vi "StageControl.vi"() -> ()   [LabVIEW 2013]
panel:
  in  "ESP Port":refnum<visa-resource-name>="COM4"
  out "Location Matrix":string[][](array[string])=[["N.D.\r\n", "N.D.\r\n", "N.D.\r\n"], ["N.D.\r\n", "N.D.\r\n", "N.D.\r\n"], ["N.D.\r\n", "N.D.\r\n", "N.D.\r\n"], ["N.D.\r\n", "N.D.\r\n", "N.D.\r\n"]]
  in  "Capture Locations":i32(listbox)=2
  in  "?":cluster{"x":string, "y":string, "z":string}={"x"="N.D.\r\n", "y"="N.D.\r\n", "z"="N.D.\r\n"}
  out "Location path":path=path "C:/Users/Fleezers/Desktop/UHR-Fleezers Instrument - Charlie/Locations.txt"
  in  "Activate Joystick":bool
  in  "VISA Clear":bool
  in  "Save":bool
  in  "Capture":bool
  in  "Goto Bottom (F7)":bool
  in  "Goto Exp (F8)":bool
  in  "Goto Top (F6)":bool
  in  "ESP ZL-Limit":string="-0.09900"
  in  "ESP ZR-Limit":string="0.09900"
  in  "error in":errorcluster
  out "X Pos":string="-0.85624\r\n"
  out "Y Pos":string="0.27735\r\n"
  out "Z Pos Pos":string="0.05734\r\n"
  out "X Motion":string="1\r\n"
  out "Y Motion":string="1\r\n"
  out "Z motion":string="1\r\n"
  out "error out":errorcluster
  in  "Axis 6":string="0.20000\r\n"
  in  "Axis 5":string="0.20000\r\n"
  in  "Axis 4":string="0.20000\r\n"
  in  "Axis 1":string="0.00500\r\n"
  in  "Axis 2":string="0.00500\r\n"
  in  "Axis 3":string="0.00500\r\n"
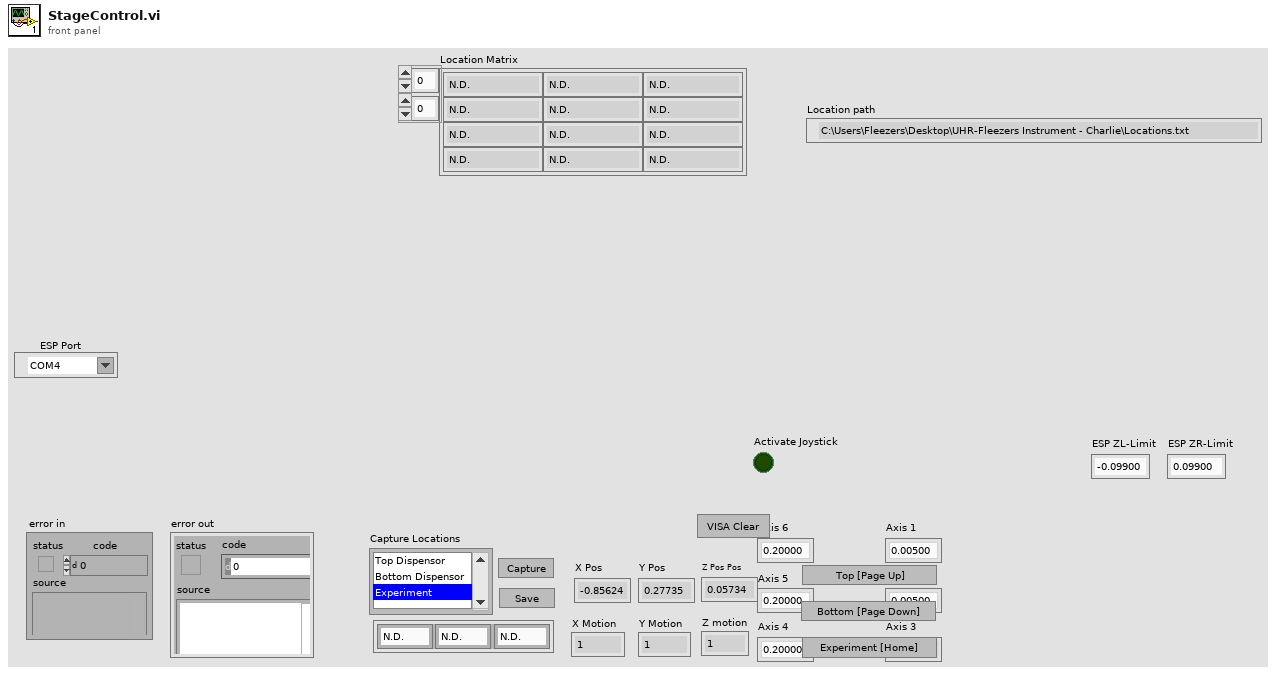
[diagram p1: front panel]
types:
  T1 = cluster{"Location Matrix[0]":string, "Location Matrix[1]":string, "Location Matrix[2]":string}
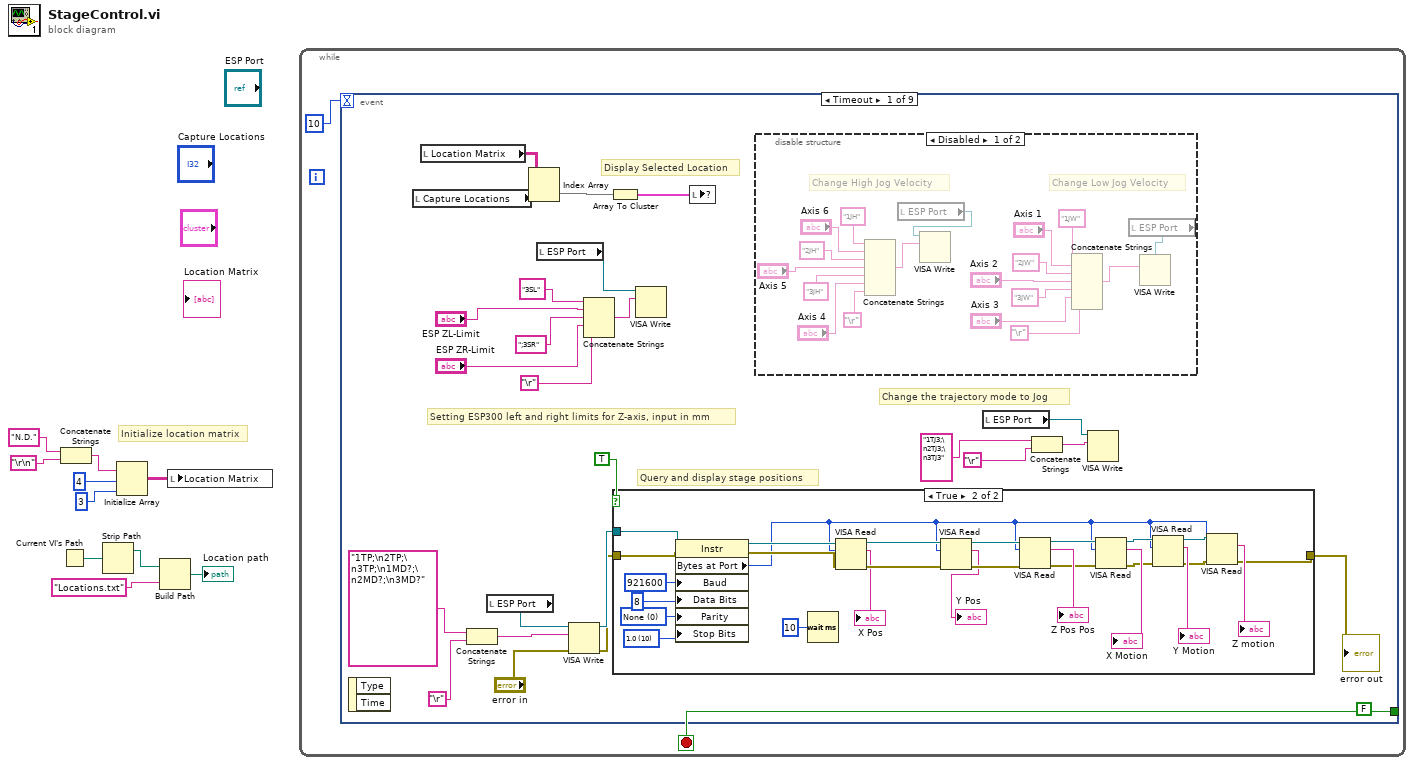
[diagram p0: block diagram]
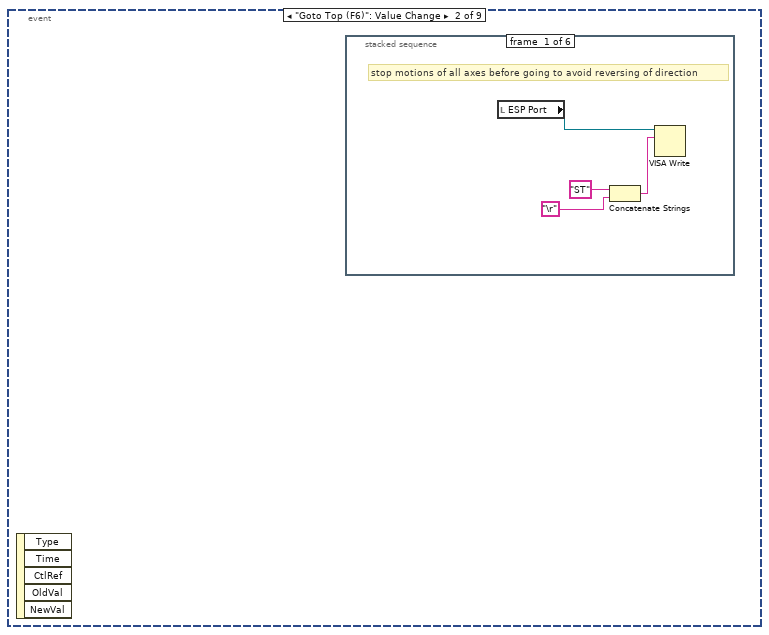
[diagram p4: hidden frame]
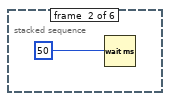
[diagram p5: hidden frame]
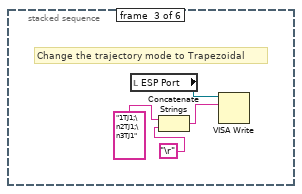
[diagram p6: hidden frame]
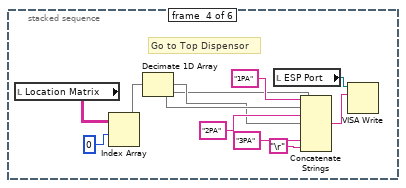
[diagram p7: hidden frame]
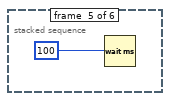
[diagram p8: hidden frame]
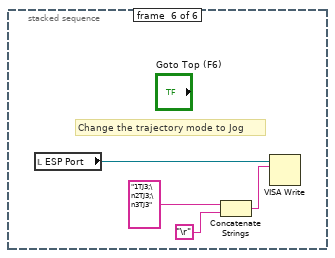
[diagram p9: hidden frame]
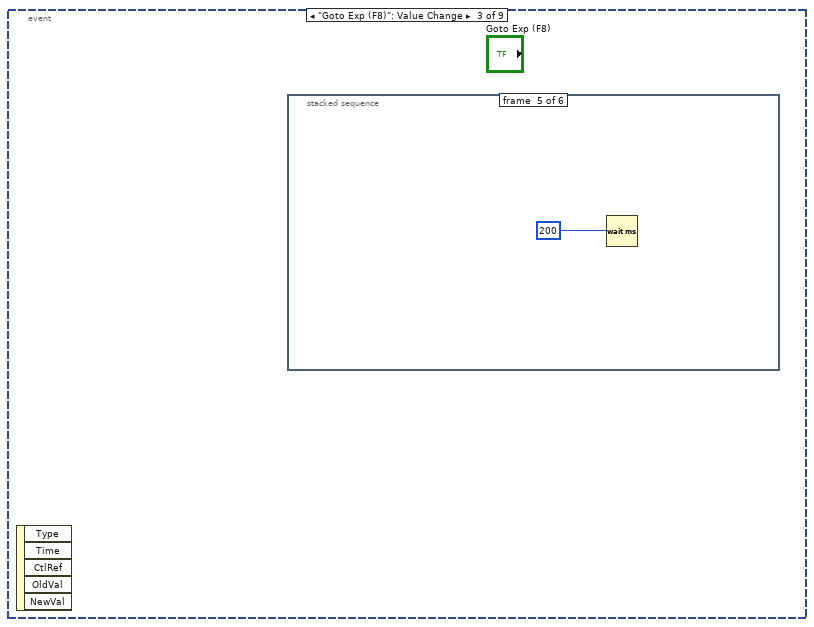
[diagram p10: hidden frame]
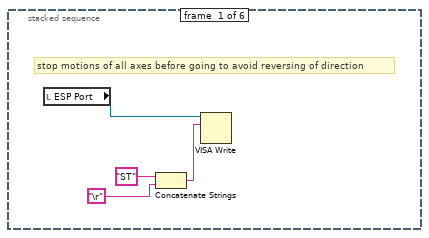
[diagram p11: hidden frame]
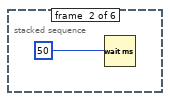
[diagram p12: hidden frame]
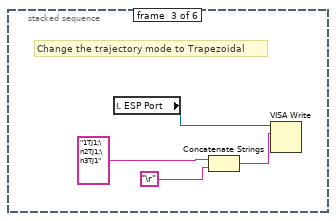
[diagram p13: hidden frame]
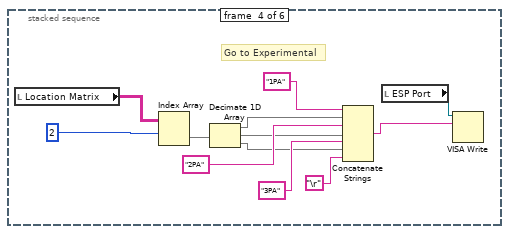
[diagram p14: hidden frame]
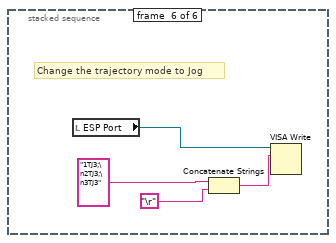
[diagram p15: hidden frame]
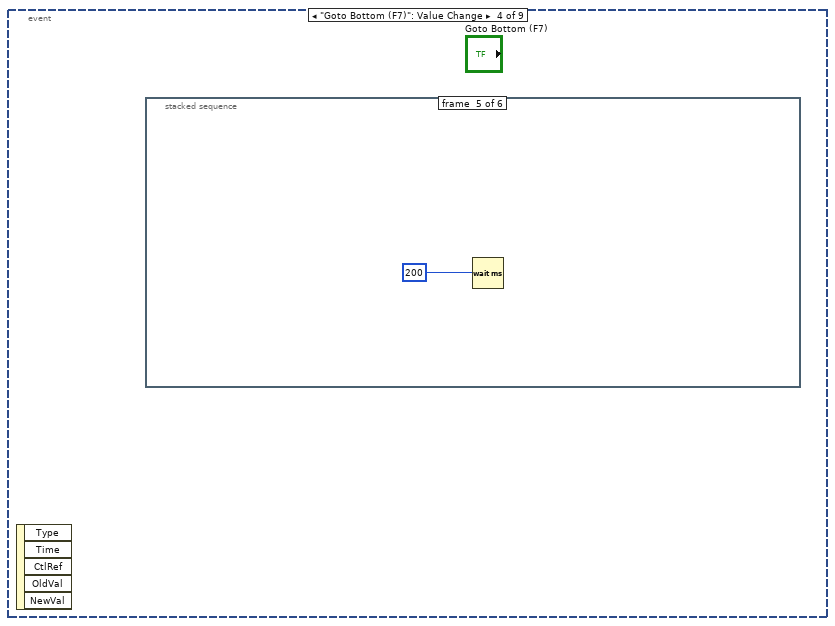
[diagram p16: hidden frame]
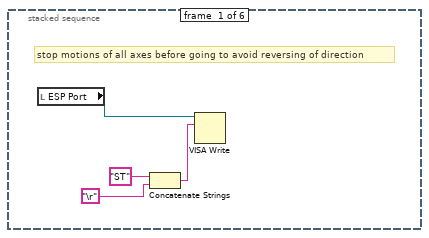
[diagram p17: hidden frame]
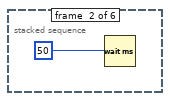
[diagram p18: hidden frame]
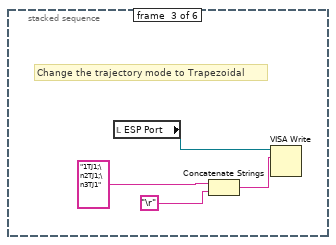
[diagram p19: hidden frame]
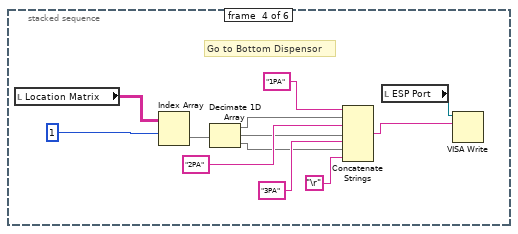
[diagram p20: hidden frame]
diagram:
  # "Initialize location matrix"
  n1 = Current VI's Path() -> (path=w10:path)
  n2 = Concatenate Strings("N.D.", "\r\n") -> (w6:string)
  n3 = Strip Path(path=w10) -> (stripped path=w9:path)  [unwired: 1 out]
  n4 = Initialize Array(w6, 4, 3) -> (w3:string[][])
  n5 = Build Path(base path=w9, name or relative path="Locations.txt") -> (appended path=→"Location path":path)
  n6 = local write "Location Matrix"(w3) -> ()
  n7 = while {
    stop <- w11 stop-if-true
    n8 = event shown="[0] Timeout" {
      selector: _ -> [_ _ _ _ _ _ _ _ _]
      dyn-events: _ -> [_ _ _ _ _ _ _ _ _]
      timeout: 10 -> [_ _ _ _ _ _ _ _ _]
      tunnel: [FALSE _ _ _ _ _ _ _ TRUE] -> w11
      event Timeout {
        # "Change the trajectory mode to Jog"
        # "Query and display stage positions"
        # "Setting ESP300 left and right limits for Z-axis, input in mm"
        # "Display Selected Location"
        n9 = event-data() -> ()  [unwired: 1 in, 2 out]
        n10 = local read "Capture Locations"() -> (w36:i32)
        n11 = local read "Location Matrix"() -> (w37:string[][])
        n12 = Concatenate Strings("1TP;\n2TP;\n3TP;\n1MD?;\n2MD?;\n3MD?" ("Substring"), "\r") -> (w20:string)
        n13 = local read "ESP Port"() -> (w23:refnum<visa-resource-name>)
        n14 = Index Array(array=w37, index (row)=w36) -> (element=w35:string[])  [unwired: 1 in]
        n15 = local read "ESP Port"() -> (w32:refnum<visa-resource-name>)
        n16 = VISA Write(VISA resource name=w23, write buffer=w20, error in (no error)="error in") -> (VISA resource name out=w21:refnum<visa-resource-name>, error out=w19:errorcluster)  [unwired: 1 out]
        n17 = Concatenate Strings("3SL" ("Substring"), "ESP ZL-Limit", ";3SR", "ESP ZR-Limit", "\r") -> (w31:string)
        n18 = Array To Cluster(array=w35) -> (cluster=w34:T1)
        n19 = case shown="True" TRUE ("Case Constant\n(See Context Help)") {
          tunnel: w21 -> [_ w75]
          tunnel: w19 -> [w56 w74]
          tunnel: [w56 w58] -> w25
          frame False {
          }
          frame True {
            w68 = u16 10 items=["1.0"=10, "1.5"=15, "2.0"=20] ("Serial Settings:Stop Bits")
            w69 = u16 0 items=["None", "Odd", "Even", "Mark", "Space"] ("Serial Settings:Parity")
            n20 = property class="Instr"(reference=w75, error in=w74, "Baud"=u32 921600 ("Serial Settings:Baud Rate"), "Data Bits"=u16 8 ("Serial Settings:Data Bits"), "Parity"=w69, "Stop Bits"=w68) -> (reference out=w73:refnum<visa-resource-name>, error out=w72:errorcluster, "Bytes at Port"=w57:u32)
            n21 = Wait (ms)(milliseconds to wait=u32 10) -> ()  [unwired: 1 out]
            n22 = VISA Read(VISA resource name=w73, byte count=w57, error in (no error)=w72) -> (VISA resource name out=w81:refnum<visa-resource-name>, read buffer=→"X Pos":string, error out=w82:errorcluster)  [unwired: 1 out]
            n23 = VISA Read(VISA resource name=w81, byte count=w57, error in (no error)=w82) -> (VISA resource name out=w79:refnum<visa-resource-name>, read buffer=→"Y Pos":string, error out=w80:errorcluster)  [unwired: 1 out]
            n24 = VISA Read(VISA resource name=w79, byte count=w57, error in (no error)=w80) -> (VISA resource name out=w67:refnum<visa-resource-name>, read buffer=→"Z Pos Pos":string, error out=w66:errorcluster)  [unwired: 1 out]
            n25 = VISA Read(VISA resource name=w67, byte count=w57, error in (no error)=w66) -> (VISA resource name out=w63:refnum<visa-resource-name>, read buffer=→"X Motion":string, error out=w64:errorcluster)  [unwired: 1 out]
            n26 = VISA Read(VISA resource name=w63, byte count=w57, error in (no error)=w64) -> (VISA resource name out=w62:refnum<visa-resource-name>, read buffer=→"Y Motion":string, error out=w60:errorcluster)  [unwired: 1 out]
            n27 = VISA Read(VISA resource name=w62, byte count=w57, error in (no error)=w60) -> (read buffer=→"Z motion":string, error out=w58:errorcluster)  [unwired: 2 out]
          }
        }
        "error out" <- w25
        n28 = VISA Write(VISA resource name=w32, write buffer=w31) -> ()  [unwired: 1 in, 3 out]
        n29 = local write item#24(w34) -> ()
        n30 = disable-structure shown="Disabled" {
          frame Disabled {
            # "Change Low Jog Velocity"
            # "Change High Jog Velocity"
            n31 = Concatenate Strings("1JH" ("Substring"), "Axis 6", "2JH" ("Substring"), "Axis 5", "3JH" ("Substring"), "Axis 4", "\r") -> (w55:string)
            n32 = local read "ESP Port"() -> (w54:refnum<visa-resource-name>)
            n33 = VISA Write(VISA resource name=w54, write buffer=w55) -> ()  [unwired: 1 in, 3 out]
            n34 = Concatenate Strings("1JW" ("Substring"), "Axis 1", "2JW" ("Substring"), "Axis 2", "3JW" ("Substring"), "Axis 3", "\r") -> (w46:string)
            n35 = local read "ESP Port"() -> (w45:refnum<visa-resource-name>)
            n36 = VISA Write(VISA resource name=w45, write buffer=w46) -> ()  [unwired: 1 in, 3 out]
          }
          frame Enabled {
          }
        }
        n37 = local read "ESP Port"() -> (w13:refnum<visa-resource-name>)
        n38 = Concatenate Strings("1TJ3;\n2TJ3;\n3TJ3" ("Substring"), "\r") -> (w14:string)
        n39 = VISA Write(VISA resource name=w13, write buffer=w14) -> ()  [unwired: 1 in, 3 out]
      }
      event "Goto Top (F6)": Value Change {
        n40 = event-data() -> ()  [unwired: 1 in, 5 out]
        n41 = stacked-sequence {
          frame #0 {
            # "stop motions of all axes before going to avoid reversing of direction"
            n42 = local read "ESP Port"() -> (w87:refnum<visa-resource-name>)
            n43 = Concatenate Strings("ST" ("Substring"), "\r") -> (w84:string)
            n44 = VISA Write(VISA resource name=w87, write buffer=w84) -> ()  [unwired: 1 in, 3 out]
          }
          frame #1 {
            n45 = Wait (ms)(milliseconds to wait=u32 50) -> ()  [unwired: 1 out]
          }
          frame #2 {
            # "Change the trajectory mode to Trapezoidal"
            n46 = local read "ESP Port"() -> (w92:refnum<visa-resource-name>)
            n47 = Concatenate Strings("1TJ1;\n2TJ1;\n3TJ1" ("Substring"), "\r") -> (w89:string)
            n48 = VISA Write(VISA resource name=w92, write buffer=w89) -> ()  [unwired: 1 in, 3 out]
          }
          frame #3 {
            # "Go to Top Dispensor"
            n49 = local read "Location Matrix"() -> (w104:string[][])
            n50 = Index Array(array=w104, index (row)=0) -> (element=w100:string[])  [unwired: 1 in]
            n51 = Decimate 1D Array(w100) -> (w98:string[], w96:string[], w94:string[])
            n52 = local read "ESP Port"() -> (w101:refnum<visa-resource-name>)
            n53 = Concatenate Strings("1PA" ("Substring"), w98, "2PA" ("Substring"), w96, "3PA" ("Substring"), w94, "\r") -> (w102:string)
            n54 = VISA Write(VISA resource name=w101, write buffer=w102) -> ()  [unwired: 1 in, 3 out]
          }
          frame #4 {
            n55 = Wait (ms)(milliseconds to wait=u32 100) -> ()  [unwired: 1 out]
          }
          frame #5 {
            # "Change the trajectory mode to Jog"
            n56 = local read "ESP Port"() -> (w109:refnum<visa-resource-name>)
            n57 = Concatenate Strings("1TJ3;\n2TJ3;\n3TJ3" ("Substring"), "\r") -> (w106:string)
            n58 = VISA Write(VISA resource name=w109, write buffer=w106) -> ()  [unwired: 1 in, 3 out]
          }
        }
      }
      event "Goto Exp (F8)": Value Change {
        n59 = event-data() -> ()  [unwired: 1 in, 5 out]
        n60 = stacked-sequence {
          frame #0 {
            # "stop motions of all axes before going to avoid reversing of direction"
            n61 = local read "ESP Port"() -> (w113:refnum<visa-resource-name>)
            n62 = Concatenate Strings("ST" ("Substring"), "\r") -> (w110:string)
            n63 = VISA Write(VISA resource name=w113, write buffer=w110) -> ()  [unwired: 1 in, 3 out]
          }
          frame #1 {
            n64 = Wait (ms)(milliseconds to wait=u32 50) -> ()  [unwired: 1 out]
          }
          frame #2 {
            # "Change the trajectory mode to Trapezoidal"
            n65 = local read "ESP Port"() -> (w118:refnum<visa-resource-name>)
            n66 = Concatenate Strings("1TJ1;\n2TJ1;\n3TJ1" ("Substring"), "\r") -> (w115:string)
            n67 = VISA Write(VISA resource name=w118, write buffer=w115) -> ()  [unwired: 1 in, 3 out]
          }
          frame #3 {
            # "Go to Experimental"
            n68 = local read "Location Matrix"() -> (w130:string[][])
            n69 = Index Array(array=w130, index (row)=2) -> (element=w126:string[])  [unwired: 1 in]
            n70 = Decimate 1D Array(w126) -> (w124:string[], w122:string[], w120:string[])
            n71 = Concatenate Strings("1PA" ("Substring"), w124, "2PA" ("Substring"), w122, "3PA" ("Substring"), w120, "\r") -> (w128:string)
            n72 = local read "ESP Port"() -> (w127:refnum<visa-resource-name>)
            n73 = VISA Write(VISA resource name=w127, write buffer=w128) -> ()  [unwired: 1 in, 3 out]
          }
          frame #4 {
            n74 = Wait (ms)(milliseconds to wait=u32 200) -> ()  [unwired: 1 out]
          }
          frame #5 {
            # "Change the trajectory mode to Jog"
            n75 = local read "ESP Port"() -> (w132:refnum<visa-resource-name>)
            n76 = Concatenate Strings("1TJ3;\n2TJ3;\n3TJ3" ("Substring"), "\r") -> (w135:string)
            n77 = VISA Write(VISA resource name=w132, write buffer=w135) -> ()  [unwired: 1 in, 3 out]
          }
        }
      }
      event "Goto Bottom (F7)": Value Change {
        n78 = event-data() -> ()  [unwired: 1 in, 5 out]
        n79 = stacked-sequence {
          frame #0 {
            # "stop motions of all axes before going to avoid reversing of direction"
            n80 = local read "ESP Port"() -> (w139:refnum<visa-resource-name>)
            n81 = Concatenate Strings("ST" ("Substring"), "\r") -> (w136:string)
            n82 = VISA Write(VISA resource name=w139, write buffer=w136) -> ()  [unwired: 1 in, 3 out]
          }
          frame #1 {
            n83 = Wait (ms)(milliseconds to wait=u32 50) -> ()  [unwired: 1 out]
          }
          frame #2 {
            # "Change the trajectory mode to Trapezoidal"
            n84 = local read "ESP Port"() -> (w144:refnum<visa-resource-name>)
            n85 = Concatenate Strings("1TJ1;\n2TJ1;\n3TJ1" ("Substring"), "\r") -> (w141:string)
            n86 = VISA Write(VISA resource name=w144, write buffer=w141) -> ()  [unwired: 1 in, 3 out]
          }
          frame #3 {
            # "Go to Bottom Dispensor"
            n87 = local read "Location Matrix"() -> (w156:string[][])
            n88 = Index Array(array=w156, index (row)=1) -> (element=w152:string[])  [unwired: 1 in]
            n89 = Decimate 1D Array(w152) -> (w150:string[], w148:string[], w146:string[])
            n90 = Concatenate Strings("1PA" ("Substring"), w150, "2PA" ("Substring"), w148, "3PA" ("Substring"), w146, "\r") -> (w154:string)
            n91 = local read "ESP Port"() -> (w153:refnum<visa-resource-name>)
            n92 = VISA Write(VISA resource name=w153, write buffer=w154) -> ()  [unwired: 1 in, 3 out]
          }
          frame #4 {
            n93 = Wait (ms)(milliseconds to wait=u32 200) -> ()  [unwired: 1 out]
          }
          frame #5 {
            # "Change the trajectory mode to Jog"
            n94 = local read "ESP Port"() -> (w158:refnum<visa-resource-name>)
            n95 = Concatenate Strings("1TJ3;\n2TJ3;\n3TJ3" ("Substring"), "\r") -> (w161:string)
            n96 = VISA Write(VISA resource name=w158, write buffer=w161) -> ()  [unwired: 1 in, 3 out]
          }
        }
      }
      event "Capture": Value Change {
        n97 = event-data() -> ()  [unwired: 1 in, 5 out]
        n98 = local read "Capture Locations"() -> (w162:i32)
        n99 = local read "Z Pos Pos"() -> (w163:string)
        n100 = local read "X Pos"() -> (w165:string)
        n101 = local read "Y Pos"() -> (w164:string)
        n102 = case shown="1" w162 {
          selector: w162 -> [w169 w176 w183 w190]
          tunnel: w165 -> [w172 w179 w186 w193]
          tunnel: w164 -> [w171 w178 w185 w192]
          tunnel: w163 -> [w170 w177 w184 w191]
          frame 0, Default {
            # "Capture Top Dispensor Location"
            n103 = local read "Location Matrix"() -> (w168:string[][])
            n104 = Build Array(w172, w171, w170) -> (w167:string[])
            n105 = Replace Array Subset(array=w168, new element=w167, index (row)=w169) -> (w166:string[][])  [unwired: 1 in]
            n106 = local write "Location Matrix"(w166) -> ()
          }
          frame 1 {
            # "Capture Bottom Dispensor Location"
            n107 = local read "Location Matrix"() -> (w175:string[][])
            n108 = Build Array(w179, w178, w177) -> (w174:string[])
            n109 = Replace Array Subset(array=w175, new element=w174, index (row)=w176) -> (w173:string[][])  [unwired: 1 in]
            n110 = local write "Location Matrix"(w173) -> ()
          }
          frame 2 {
            # "Capture Experimental Region Location"
            n111 = local read "Location Matrix"() -> (w182:string[][])
            n112 = Build Array(w186, w185, w184) -> (w181:string[])
            n113 = Replace Array Subset(array=w182, new element=w181, index (row)=w183) -> (w180:string[][])  [unwired: 1 in]
            n114 = local write "Location Matrix"(w180) -> ()
          }
          frame 3 {
            # "Capture Other Location"
            n115 = local read "Location Matrix"() -> (w189:string[][])
            n116 = Build Array(w193, w192, w191) -> (w188:string[])
            n117 = Replace Array Subset(array=w189, new element=w188, index (row)=w190) -> (w187:string[][])  [unwired: 1 in]
            n118 = local write "Location Matrix"(w187) -> ()
          }
        }
      }
      event "Save": Value Change {
        # "reshape Location Matrix to 1-D array to write"
        n119 = event-data() -> ()  [unwired: 1 in, 5 out]
        n120 = local read "Location Matrix"() -> (w197:string[][])
        n121 = local read "Location path"() -> (w194:path)
        n122 = Reshape Array(w197, 12) -> (w195:string[])
        n123 = Write to Text File(file (use dialog)=w194, text=w195) -> ()  [unwired: 2 in, 3 out]
      }
      event "VISA Clear": Value Change {
        n124 = event-data() -> ()  [unwired: 1 in, 5 out]
        n125 = local read "ESP Port"() -> (w198:refnum<visa-resource-name>)
        n126 = VISA Clear(VISA resource name=w198) -> ()  [unwired: 1 in, 2 out]
      }
      event "Activate Joystick": Value Change {
        # "Change the trajectory mode to Jog"
        n127 = event-data() -> ()  [unwired: 1 in, 5 out]
        n128 = disable-structure shown="Disabled" {
          frame Disabled {
            n129 = case shown="True" "Activate Joystick" {
              frame False {
              }
              frame True {
                # "Change the trajectory mode to Jog"
                n130 = local read "ESP Port"() -> (w207:refnum<visa-resource-name>)
                n131 = Concatenate Strings("1TJ3;\n2TJ3;\n3TJ3" ("Substring"), "\r") -> (w204:string)
                n132 = VISA Write(VISA resource name=w207, write buffer=w204) -> ()  [unwired: 1 in, 3 out]
              }
            }
          }
          frame Enabled {
          }
        }
        n133 = local read "ESP Port"() -> (w199:refnum<visa-resource-name>)
        n134 = Concatenate Strings("1TJ3;\n2TJ3;\n3TJ3" ("Substring"), "\r") -> (w202:string)
        n135 = VISA Write(VISA resource name=w199, write buffer=w202) -> ()  [unwired: 1 in, 3 out]
      }
      event #8 (no event record) {
        n136 = event-data() -> ()  [unwired: 1 in, 5 out]
      }
    }
  }
